vi "RGBtoColor.vi"(1 "Blue":i32, 2 "Green":i32, 3 "Red":i32) -> (0 "Color":i32)   [LabVIEW 2010]
doc: "Convert red, blue and green values to a color value, that is used by the IC Imaging Control OverlayBitmap methods."
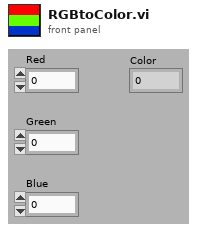
[diagram p1: front panel]
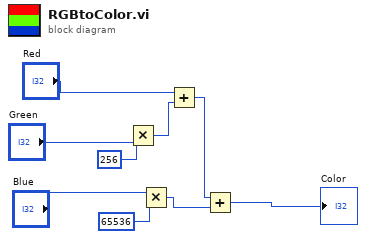
[diagram p0: block diagram]
diagram:
  n1 = Multiply(x="Green", y=256) -> (x*y=w4:i32)
  n2 = Multiply(x="Blue", y=65536) -> (x*y=w9:i32)
  n3 = Add(x="Red", y=w4) -> (x+y=w5:i32)
  n4 = Add(x=w5, y=w9) -> (x+y=→"Color":i32)
